vi "Cleanup Session.vi"(8 "error in":errorcluster, 11 "Plugin in":refnum<class "StreamReader.lvclass">) -> (0 "error out":errorcluster, 3 "Plugin out":refnum<class "StreamReader.lvclass">)   [LabVIEW 2024, in "StreamReader.lvlib" / "StreamReader.lvclass"]
uses:
  StreamReader.lvclass
  StreamReader.lvclass/StreamReader.ctl
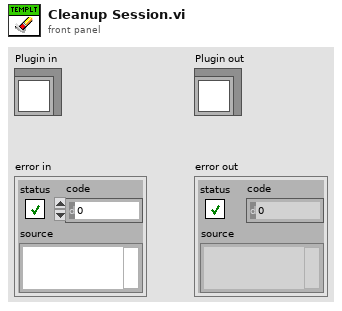
[diagram p1: front panel]
types:
  T1 = typedef "StreamReader.lvlib/StreamReader.lvclass/StreamReader Parameters.ctl" = cluster{"Writer IP Address":string, "Timeout":i32, "Buffer Size":i32, "Reader endpoint":refnum<k21>, "Channel Names":string[]}
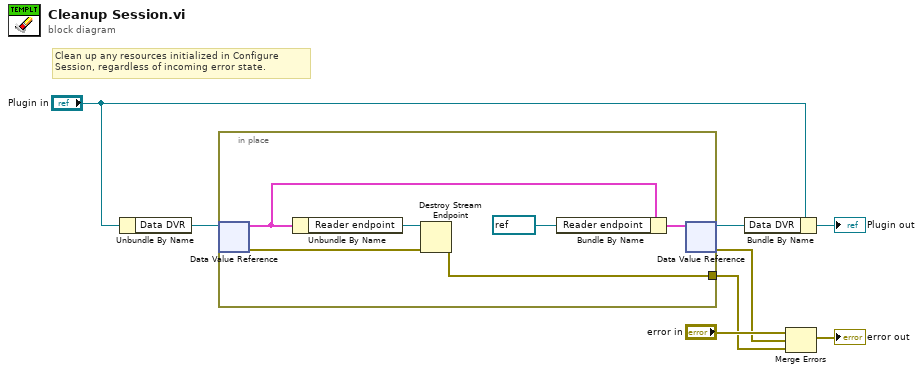
[diagram p0: block diagram]
diagram:
  # "Clean up any resources initialized in Configure Session, regardless of incoming error state."
  n1 = Unbundle By Name("Plugin in") -> ("Data DVR"=w6:refnum<data-value>)
  n2 = in-place {
    in-place-border: [w9] -> w1
    n3 = in-place-dvr #1(w6) -> (w12:T1, w13:errorcluster)
    n4 = Unbundle By Name(w12) -> ("Reader endpoint"=w14:refnum<k21>)
    n5 = Destroy Stream Endpoint(8:w13, 11:w14) -> (0:w9:errorcluster)
    n6 = Bundle By Name(cluster=w12, "Reader endpoint"=refnum<k21> refnum) -> (w10:T1)
    n7 = in-place-dvr #1(w10) -> (w5:refnum<data-value>, w2:errorcluster)
  }
  n8 = Bundle By Name(cluster="Plugin in", "Data DVR"=w5) -> (→"Plugin out":refnum<class "StreamReader.lvclass">)
  n9 = Merge Errors("error in", w2, w1) -> (→"error out":errorcluster)
